vi "Current Loop - NI 9505 (RT).vi"() -> ()   [LabVIEW 2012]
doc: "This VI shows an example of how to implement a current loop for use with the NI 9505. The VI consists of a closed loop PI system with PWM generation and error monitoring. The desired load current can be set and the loop will monitor the actual current and adjust the PWM duty cycle until the desired current is reached."
uses:
  <vilib>/LabVIEW Targets/FPGA/cRIO/cRIO-9505/controls.llb/_nicrio_cRIO-9505_DriveStatus.ctl
  <vilib>/FPGAPlugInAG/cRIO-9075/niLvFpga_Open_cRIO-9075.vi
  <vilib>/Utility/error.llb/Error Cluster From Error Code.vi
  <vilib>/rvi/errors/niLvFpgaAdjustHostInterfaceError.vi
  <vilib>/FPGAPlugInAG/cRIO-9075/niLvFpga_Close_cRIO-9075.vi
  <vilib>/rvi/interface/nirviOpenFPGA/nirviOpenFPGA.xnode
  FPGA Bitfiles/CurrentLoop-NI95_FPGATarget_CurrentLoop-NI95_7d7WRMxQUkw.lvbitx
  Current Loop - NI 9505 (FPGA).vi
  <vilib>/rvi/interface/nirviReadWriteControl/nirviReadWriteControl.xnode
  <vilib>/rvi/interface/nirviCloseFPGA/nirviCloseFPGA.xnode
  NiFpgaLv.dll
panel:
  out "Measured Force (N)":fxp<+,39,10>
  in  "Command Force (N)":fxp<+,16,6>
  in  "Enable Drive":bool
  out "error out":errorcluster
  in  "Current Loop Rate (usec)":u32=50
  in  "Current PI Gains":T1={"Proportional Gain"=20, "Integral Gain"=10, "Derivative Gain"=0}
  in  "Current Limit (Amps)":dbl=1.0 min=0.0 max=12.0
  in  "Drive Direction":enum16{"Clockwise", "Counterclockwise"}(ring)
  in  "stop":bool
  out "Drive Status":T2=enum."Disabled"
  out "Measured Current (Amps)":dbl
  in  "Current Setpoint (Amps)":dbl min=0.0 max=12.0
  # "VI Execution\n1. Set Current Limit (Amps) to a value appropriate for your load.\n2. The Current PI Gains should not need to be changed from the default values.\n2. Set Drive Direction to the desired value.\n3. Run the VI.\n4. Adjust Current Setpoint (Amps) to vary the current in the load. Maximum setpoint is 12 A. However, the module is only rated for 5 A continuous current at 40 ºC or below. 12 A is the allowable peak current. Refer to the \"NI 9505 Operating Instructions and Specifications\" for complete specifications.\n5. Measured Current (Amps) returns the actual load current."
  # "Current Loop Parameters"
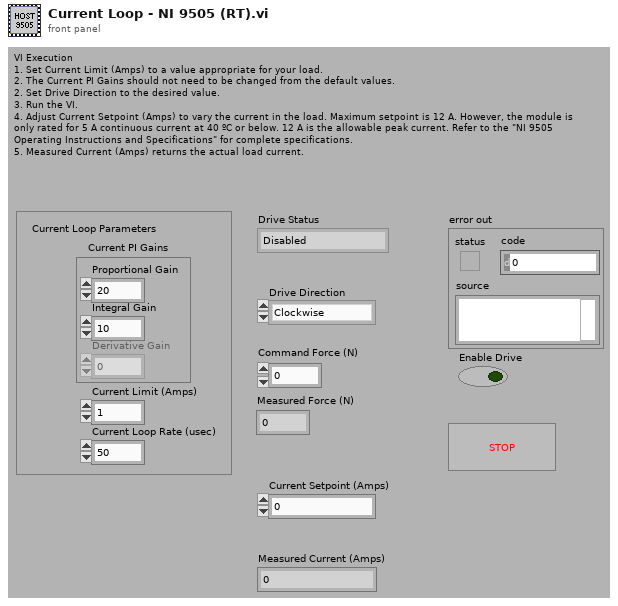
[diagram p1: front panel]
types:
  T1 = cluster{"Proportional Gain":i16, "Integral Gain":i16, "Derivative Gain":i16}
  T2 = typedef "_nicrio_cRIO-9505_DriveStatus.ctl" = enum8{"Enabled", "Disabled", "Disabled by Drive Fault", "Disabled by Temp. Fault", "Disabled by E-Stop", "Unknown"}
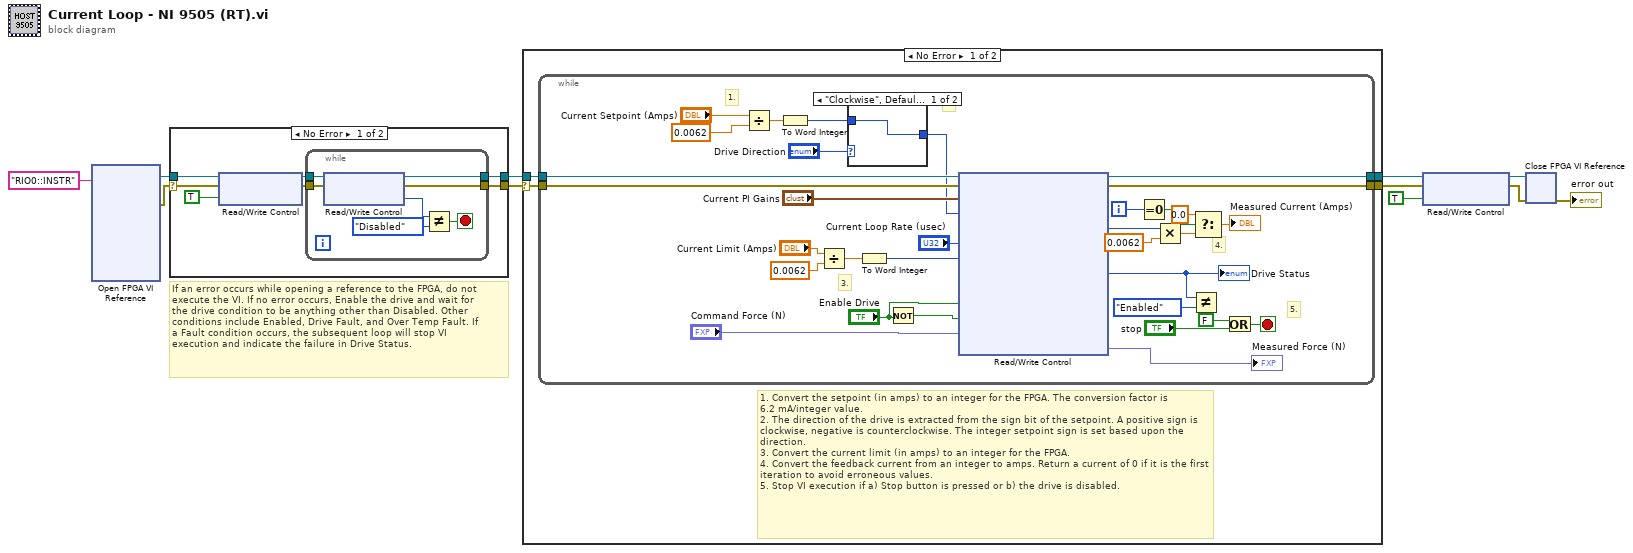
[diagram p0: block diagram]
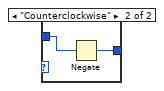
[diagram p2: hidden frame]
diagram:
  # "If an error occurs while opening a reference to the FPGA, do not\nexecute the VI. If no error occurs, Enable the drive and wait for\nthe drive condition to be anything other than Disabled. Other\nconditions include Enabled, Drive Fault, and Over Temp Fault. If\na Fault condition occurs, the subsequent loop will stop VI\nexecution and indicate the failure in Drive Status."
  n1 = xnode "Open FPGA VI Reference"("resource name"="RIO0::INSTR") -> ("FPGA VI Reference Out"=w4:refnum<k20>, "error out"=w3:errorcluster)  [unwired: 1 in]
  n2 = case shown="No Error" w3 {
    selector: w3 -> [w13 w26]
    tunnel: w4 -> [w16 w27]
    tunnel: [w18 w27] -> w6
    tunnel: [w12 w26] -> w5
    frame No Error {
      n3 = xnode "Read/Write Control"("FPGA VI Reference In"=w16, "error in"=w13, "Enable Drive"=TRUE) -> ("FPGA VI Reference Out"=w15:refnum<k20>, "error out"=w14:errorcluster)
      n4 = while {
        tunnel: [w25] -> w18
        tunnel: w15 -> [w21]
        tunnel: w14 -> [w22]
        tunnel: [w19] -> w12
        stop <- w20 stop-if-true
        n5 = xnode "Read/Write Control"("FPGA VI Reference In"=w21, "error in"=w22) -> ("FPGA VI Reference Out"=w25:refnum<k20>, "error out"=w19:errorcluster, "Drive Status"=w24:T2)
        n6 = Not Equal?(x=w24, y=_nicrio_cRIO-9505_DriveStatus."Disabled") -> (x != y?=w20:bool)
      }
    }
    frame Error {
      # "Error occurred. Do not run."
    }
  }
  n7 = case shown="No Error" w5 {
    selector: w5 -> [w28 w67]
    tunnel: [w31 w68] -> w11
    tunnel: [w30 w67] -> w10
    tunnel: w6 -> [w29 w68]
    frame No Error {
      # "1. Convert the setpoint (in amps) to an integer for the FPGA. The conversion factor is \n6.2 mA/integer value.\n2. The direction of the drive is extracted from the sign bit of the setpoint. A positive sign is clockwise, negative is counterclockwise. The integer setpoint sign is set based upon the direction.\n3. Convert the current limit (in amps) to an integer for the FPGA.\n4. Convert the feedback current from an integer to amps. Return a current of 0 if it is the first iteration to avoid erroneous values.\n5. Stop VI execution if a) Stop button is pressed or b) the drive is disabled."
      n8 = while {
        tunnel: w29 -> [w63]
        tunnel: [w61] -> w31
        tunnel: w28 -> [w62]
        tunnel: [w60] -> w30
        i -> [w39]
        stop <- w46 stop-if-true
        # "5."
        # "4."
        # "3."
        # "2."
        # "1."
        n9 = Divide(x="Current Setpoint (Amps)", y=0.0062) -> (x/y=w54:dbl)
        n10 = To Word Integer(number=w54) -> (16bit integer=w50:i16)
        n11 = Divide(x="Current Limit (Amps)", y=0.0062) -> (x/y=w53:dbl)
        n12 = case shown="\"Clockwise\", Default" "Drive Direction" {
          tunnel: w50 -> [w64 w66]
          tunnel: [w64 w65] -> w49
          frame "Clockwise", Default {
          }
          frame "Counterclockwise" {
            n13 = Negate(x=w66) -> (-x=w65:i16)
          }
        }
        n14 = To Word Integer(number=w53) -> (16bit integer=w52:i16)
        n15 = Not(x="Enable Drive") -> (.not. x?=w35:bool)
        n16 = xnode "Read/Write Control"("FPGA VI Reference In"=w63, "error in"=w62, "Current PI gains"="Current PI Gains", "Current Setpoint"=w49, "Current Loop Rate (usec)"="Current Loop Rate (usec)", "Current Limit"=w52, "Enable Drive"="Enable Drive", "Disable Drive"=w35, "Command Force (N)"="Command Force (N)") -> ("FPGA VI Reference Out"=w61:refnum<k20>, "error out"=w60:errorcluster, "Current Feedback"=w41:i16, "Drive Status"=w48:T2, "Measured Force (N)"=→"Measured Force (N)":fxp<+,39,10>)  [unwired: 1 out]
        "Drive Status" <- w48
        n17 = Equal To 0?(x=w39) -> (x = 0?=w38:bool)
        n18 = Multiply(x=w41, y=0.0062) -> (x*y=w43:dbl)
        n19 = Not Equal?(x=w48, y=_nicrio_cRIO-9505_DriveStatus."Enabled") -> ()  [unwired: 1 out]
        n20 = Select(t=0.0, s=w38, f=w43) -> (s? t:f=→"Measured Current (Amps)":dbl)
        n21 = Or(x=FALSE, y="stop") -> (x .or. y?=w46:bool)
      }
    }
    frame Error {
      # "Error occurred. Do not run."
    }
  }
  n22 = xnode "Read/Write Control"("FPGA VI Reference In"=w11, "error in"=w10, "Disable Drive"=TRUE) -> ("FPGA VI Reference Out"=w8:refnum<k20>, "error out"=w7:errorcluster)
  n23 = xnode "Close FPGA VI Reference"("FPGA VI Reference In"=w8, "error in"=w7) -> ("error out"=→"error out":errorcluster)
